vi "readVoltage.vi"(1 "Channel Index":i32 min=0 max=15) -> (0 "Voltage":dbl)   [LabVIEW 2011]
uses:
  globals.vi
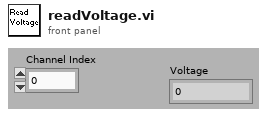
[diagram p1: front panel]
types:
  T1 = cluster{"Relay Card Slots":cluster{"Card 1":u16, "Card 2":u16, "Card 3":u16, "Card 4":u16, "Card 5":u16}, "A/D Card Slots":cluster{"Scanner":u16, "High-Speed A/D":u16, "Timer":u16}, "D/A Cards":cluster{"Quad (10-bit) D/A Card Slots":cluster{"Card 1":u16, "Card 2":u16, "Card 3":u16, "Card 4":u16, "Card 5":u16}, "Single (12-bit) D/A Card Slot":cluster{"Card 6":u16}}}
  T2 = cluster{"Scanner":u16, "High-Speed A/D":u16, "Timer":u16}
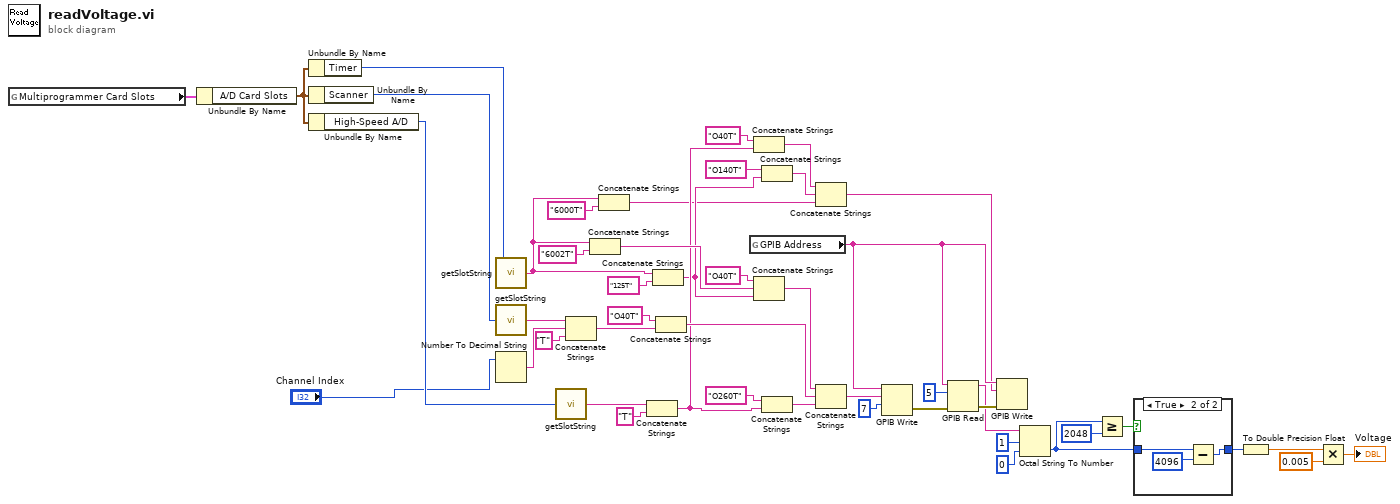
[diagram p0: block diagram]
diagram:
  n1 = global read "globals.vi" "Multiprogrammer Card Slots"() -> (w6:T1)
  n2 = Unbundle By Name(w6) -> ("A/D Card Slots"=w3:T2)
  n3 = Unbundle By Name(w3) -> ("Timer"=w5:u16)
  n4 = Unbundle By Name(w3) -> ("Scanner"=w4:u16)
  n5 = Unbundle By Name(w3) -> ("High-Speed A/D"=w2:u16)
  n6 = call "getSlotString.vi"("Slot"=w5) -> ("string"=w12:string)
  n7 = call "getSlotString.vi"("Slot"=w4) -> ("string"=w27:string)
  n8 = Number To Decimal String(number="Channel Index") -> (decimal integer string=w26:string)  [unwired: 1 out]
  n9 = call "getSlotString.vi"("Slot"=w2) -> ("string"=w22:string)
  n10 = Concatenate Strings(w27, w26, "T" ("string")) -> (w25:string)
  n11 = Concatenate Strings(w12, "6002T" ("data")) -> (w29:string)
  n12 = Concatenate Strings(w12, "6000T" ("data")) -> (w8:string)
  n13 = Concatenate Strings(w22, "T" ("string")) -> (w16:string)
  n14 = Concatenate Strings(w12, "125T" ("data")) -> (w13:string)
  n15 = Concatenate Strings("O40T" ("data"), w25) -> (w19:string)
  n16 = global read "globals.vi" "GPIB Address"() -> (w33:string)
  n17 = Concatenate Strings("O40T" ("data"), w16) -> (w10:string)
  n18 = Concatenate Strings("O40T" ("data"), w29, w13) -> (w20:string)
  n19 = Concatenate Strings("O140T" ("data"), w13) -> (w9:string)
  n20 = Concatenate Strings("O260T" ("string"), w16) -> (w18:string)
  n21 = Concatenate Strings(w10, w9, w8) -> (w7:string)
  n22 = Concatenate Strings(w20, w19, w18) -> (w36:string)
  n23 = GPIB Write(0:w33, 1:w36, 2:i16 7 ("mode (0)")) -> (6:w47:errorcluster)  [unwired: 1 in, 2 out]
  n24 = GPIB Read(0:w33, 1:5 ("byte count"), 3:w47) -> (5:w44:string, 7:w46:errorcluster)  [unwired: 3 out]
  n25 = GPIB Write(0:w33, 1:w7, 3:w46) -> ()  [unwired: 4 out]
  n26 = Octal String To Number(2:0 ("default (0 U32)"), 3:1 ("offset"), 4:w44) -> (0:w38:i32)  [unwired: 1 out]
  n27 = Greater Or Equal?(x=w38, y=2048) -> (x >= y?=w39:bool)
  n28 = case shown="True" w39 {
    tunnel: w38 -> [w48 w49]
    tunnel: [w48 w51] -> w37
    frame False {
    }
    frame True {
      n29 = Subtract(x=w49, y=4096 ("x")) -> (x-y=w51:i32)
    }
  }
  n30 = To Double Precision Float(number=w37) -> (double precision float=w43:dbl)
  n31 = Multiply(x=w43, y=0.005) -> (x*y=→"Voltage":dbl)
